vi "Calculate Frame Timing.vi"(9 "estimated next frame start timestamp":u64, 10 "frame start timestamp":u64, 11 "desired frame rate (fps)":dbl) -> (2 "actual next frame start timestamp":u64, 3 "actual frame rate (fps)":dbl)   [LabVIEW 2023, in "GettingStarted_Gen_148X_Host.lvlib"]
uses:
  GettingStarted_Gen_148X_Host.lvlib
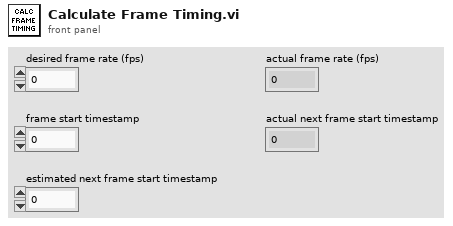
[diagram p1: front panel]
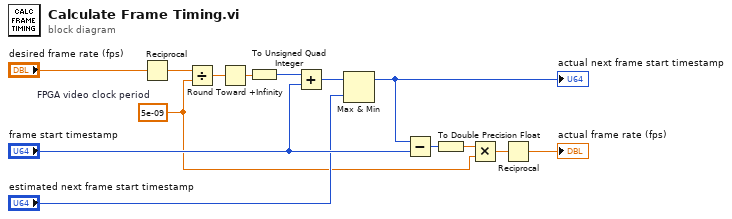
[diagram p0: block diagram]
diagram:
  w1 = 5e-09  # FPGA video clock period
  n1 = Reciprocal(x="desired frame rate (fps)") -> (1/x=w5:dbl)
  n2 = Divide(x=w5, y=w1) -> (x/y=w3:dbl)
  n3 = Round Toward +Infinity(x=w3) -> (ceil(x): smallest int >= x=w4:dbl)
  n4 = To Unsigned Quad Integer(1:w4) -> (0:w7:u64)
  n5 = Add(x=w7, y="frame start timestamp") -> (x+y=w8:u64)
  n6 = Max & Min(x=w8, y="estimated next frame start timestamp") -> (max(x,y)=w9:u64)  [unwired: 1 out]
  "actual next frame start timestamp" <- w9
  n7 = Subtract(x=w9, y="frame start timestamp") -> (x-y=w11:u64)
  n8 = To Double Precision Float(number=w11) -> (double precision float=w12:dbl)
  n9 = Multiply(x=w12, y=w1) -> (x*y=w13:dbl)
  n10 = Reciprocal(x=w13) -> (1/x=→"actual frame rate (fps)":dbl)
